vi "Inverter_MAIN.vi"() -> ()   [LabVIEW 2020]
uses:
  controls/INV_test results.ctl
  controls/Inverter_step_type.ctl
  MPB/controls/test control_bools.ctl
  MPB/controls/from_PLC.ctl
  MPB/controls/to_PLC.ctl
  MPB/controls/test_control.ctl
  controls/Inverter_step_array.ctl
  controls/Inverter_step.ctl
  MPB/controls/data type.ctl
  MPB/controls/write_read.ctl
  Hardware Drivers/Keysight E3633 DC PS/dc ps control.ctl
  3b758781-4fb9-4e00-a9b5-a1315665c223.vi
  a98f73de-f23d-4de7-99eb-8fa248b25b7f.vi
panel:
  in  "Test Station":T1
  in  "PLC":T2
  in  "test control":T3
  out "test results":T4={"test pass"=FALSE, "step_type"=enum."prompt", "value"=0.0, "step description"="", "error"={"status"=FALSE, "code"=0, "source"=""}, "save results"=FALSE}
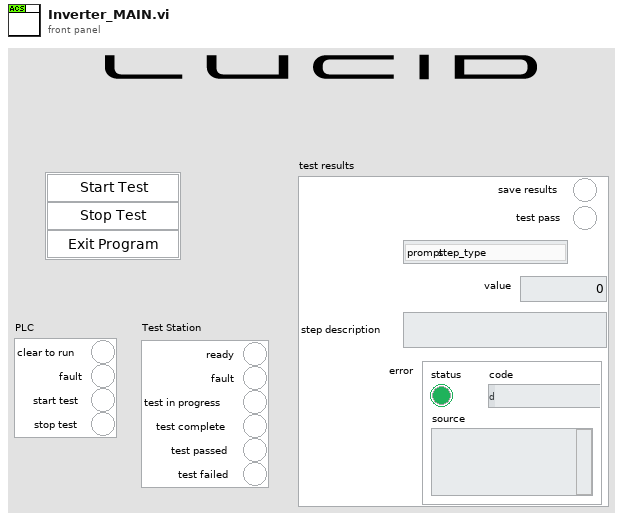
[diagram p1: front panel]
types:
  T1 = typedef "to_PLC.ctl" = cluster{"ready":bool, "fault":bool, "test in progress":bool, "test complete":bool, "test passed":bool, "test failed":bool}
  T2 = typedef "from_PLC.ctl" = cluster{"clear to run":bool, "fault":bool, "start test":bool, "stop test":bool}
  T3 = typedef "test control_bools.ctl" = cluster{"Exit Program":bool, "Stop Test":bool, "Start Test":bool}
  T4 = typedef "INV_test results.ctl" = cluster{"test pass":bool, "step_type":T5, "value":dbl, "step description":string, "error":errorcluster, "save results":bool}
  T5 = typedef "Inverter_step_type.ctl" = enum16{"default", "prompt", "init_12V_power_supply", "12V_power supply on_off", "write_PLC", "read_PLC", "DAQ_Read", "DAQ_Write", "run .bat file", "display_version", "set flow rate", "init_chroma", "set_chroma_V", "set_chroma_ramp", "wait (sec)", "end_test", "record_pass_fail"}
  T6 = typedef "test_control.ctl" = enum16{"Start Test", "Stop Test", "Ready", "Exit Program"}
  T7 = typedef "Inverter_step_array.ctl" = T8[]
  T8 = typedef "Inverter_step.ctl" = cluster{"step_description (prompt)":string, "save results":bool, "step_type":T5, "Step_name":string, "bool":bool[], "data_unit":T9, "dbl":dbl[], "I32":i32[], "string":string[]}
  T9 = typedef "data type.ctl" = enum16{"bool", "string", "I32", "DBL"}
  T10 = cluster{"queue out":refnum<queue>, "queue out":refnum<queue>, "queue out":refnum<queue>}
  T11 = cluster{"Inverter Step Array":T7, "error constant":errorcluster}
  T12 = typedef "dc ps control.ctl" = enum16{"init", "config output", "config OVP", "config current limit", "output on_off", "read output", "self test", "close"}
  T13 = typedef "write_read.ctl" = enum16{"write", "read"}
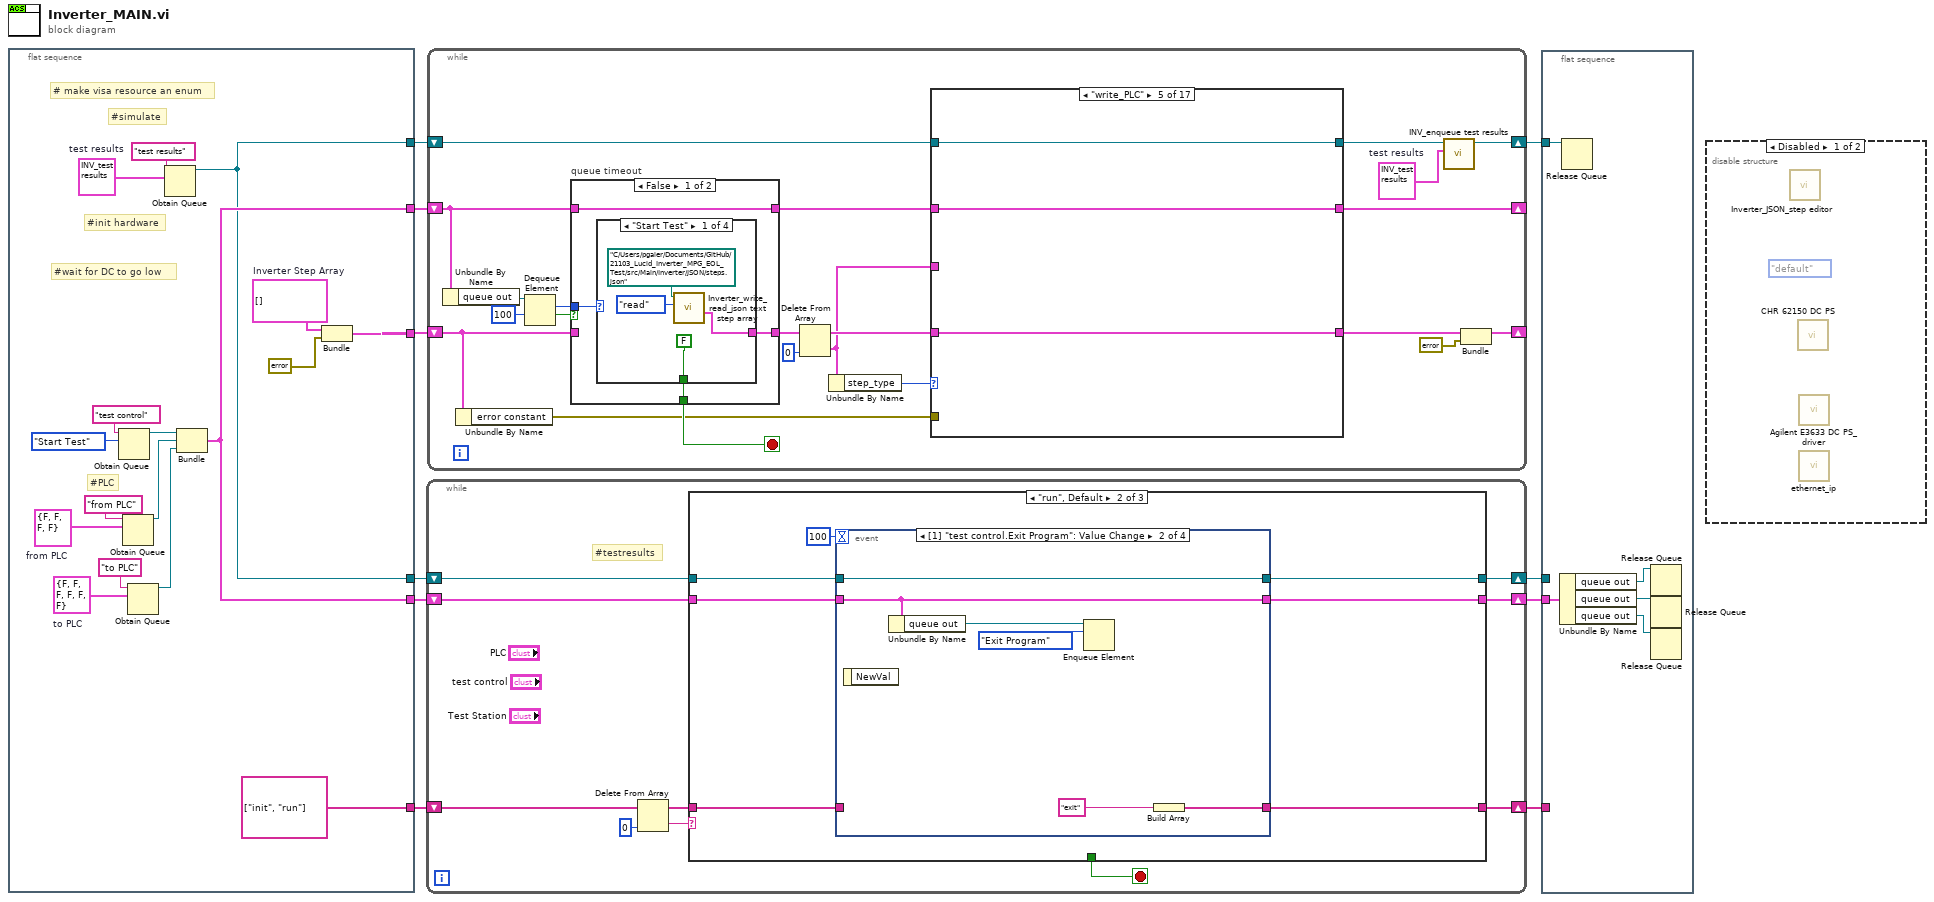
[diagram p0: block diagram]
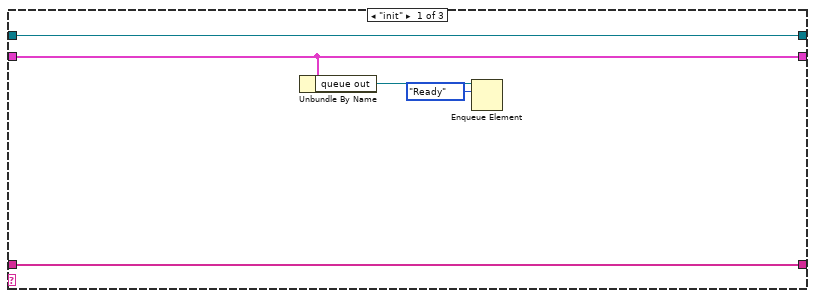
[diagram p3: hidden frame]
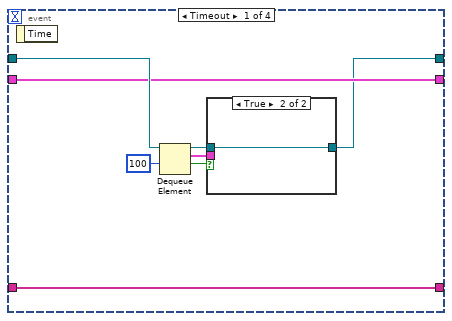
[diagram p4: hidden frame]
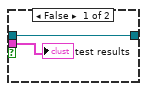
[diagram p5: hidden frame]
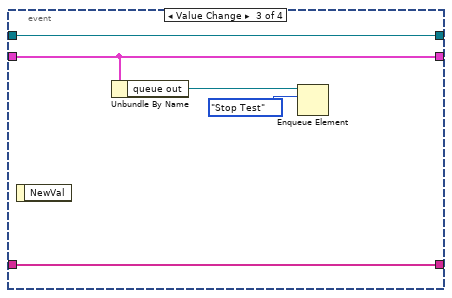
[diagram p6: hidden frame]
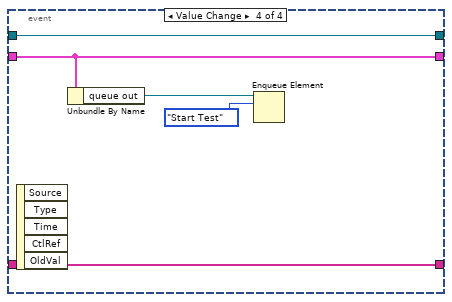
[diagram p7: hidden frame]
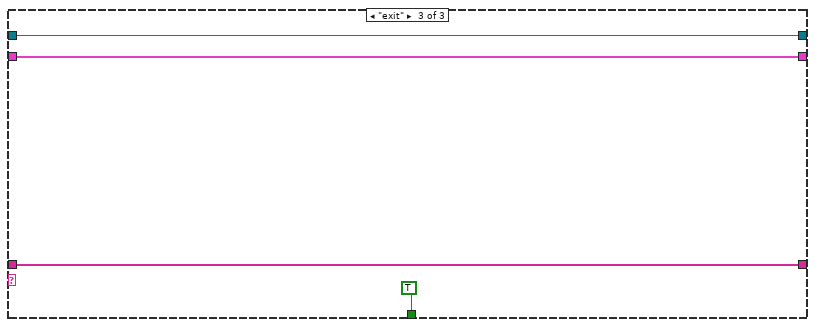
[diagram p8: hidden frame]
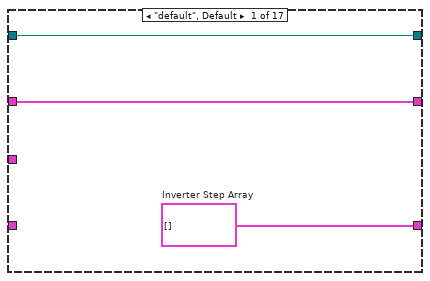
[diagram p9: hidden frame]
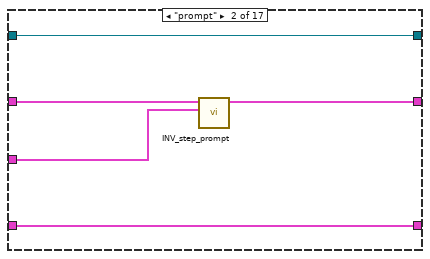
[diagram p10: hidden frame]
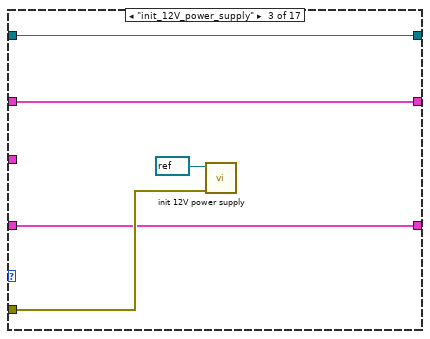
[diagram p11: hidden frame]
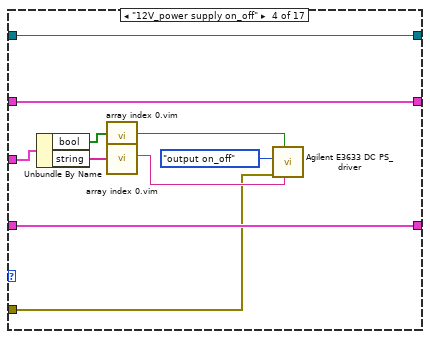
[diagram p12: hidden frame]
diagram:
  n1 = flat-sequence {
    tunnel: [w14] -> w10
    tunnel: [string[] ["init", "run"]] -> w9
    tunnel: [w15] -> w8
    tunnel: [w15] -> w7
    tunnel: [w22] -> w6
    tunnel: [w22] -> w5
    frame #0 {
      w11 = T7 []  # Inverter Step Array
      w23 = T1 {"ready"=FALSE, "fault"=FALSE, "test in progress"=FALSE, "test complete"=FALSE, "test passed"=FALSE, "test failed"=FALSE}  # to PLC
      w24 = T2 {"clear to run"=FALSE, "fault"=FALSE, "start test"=FALSE, "stop test"=FALSE}  # from PLC
      w26 = T4 {"test pass"=FALSE, "step_type"=enum."prompt", "value"=0.0, "step description"="", "error"={"status"=FALSE, "code"=0, "source"=""}, "save results"=FALSE}  # test results
      # "#init hardware"
      # "#wait for DC to go low"
      # "#PLC"
      # "#simulate"
      # "# make visa resource an enum"
      n2 = Obtain Queue(name (unnamed)="test control", element data type=test_control."Start Test" ("test control")) -> (queue out=w25:refnum<queue>)  [unwired: 3 in, 2 out]
      n3 = Obtain Queue(name (unnamed)="from PLC", element data type=w24) -> (queue out=w17:refnum<queue>)  [unwired: 3 in, 2 out]
      n4 = Obtain Queue(name (unnamed)="to PLC", element data type=w23) -> (queue out=w16:refnum<queue>)  [unwired: 3 in, 2 out]
      n5 = Obtain Queue(name (unnamed)="test results", element data type=w26) -> (queue out=w15:refnum<queue>)  [unwired: 3 in, 2 out]
      n6 = Bundle("queue out"=w25, "queue out"=w17, "queue out"=w16) -> (w22:T10)  [unwired: 1 in]
      n7 = Bundle("Inverter Step Array"=w11, "error constant"=errorcluster {"status"=FALSE, "code"=0, "source"=""}) -> (w14:T11)  [unwired: 1 in]
    }
  }
  n8 = while {
    shift-right: [w34] -> w4
    shift-left: w9 -> [w36]
    shift-right: [w29] -> w3
    shift-left: w7 -> [w32]
    shift-right: [w28] -> w2
    shift-left: w6 -> [w31]
    stop <- w30 stop-if-true
    # "#testresults"
    n9 = Delete From Array(array=w36, index=0) -> (deleted portion=w35:string, array with subset deleted=w33:string[])  [unwired: 1 in]
    n10 = case shown="\"run\", Default" w35 {
      tunnel: [w42 w49 w80] -> w34
      tunnel: w33 -> [w42 w48 w80]
      tunnel: w32 -> [w41 w47 w79]
      tunnel: w31 -> [w39 w46 w78]
      tunnel: [_ _ TRUE] -> w30
      tunnel: [w41 w45 w79] -> w29
      tunnel: [w39 w44 w78] -> w28
      frame "init" {
        n11 = Unbundle By Name(w39) -> ("queue out"=w38:refnum<queue>)
        n12 = Enqueue Element(queue=w38, element=test_control."Ready" ("test control")) -> ()  [unwired: 2 in, 3 out]
      }
      frame "run", Default {
        n13 = event shown="[1] \"test control.Exit Program\": Value Change" {
          selector: _ -> [_ _ _ _]
          dyn-events: _ -> [_ _ _ _]
          timeout: 100 -> [_ _ _ _]
          tunnel: w48 -> [w57 _ w71 w76]
          tunnel: [w57 w64 w71 w76] -> w49
          tunnel: w47 -> [w56 w66 w70 w75]
          tunnel: w46 -> [w55 w61 w67 w72]
          tunnel: [w52 w66 w70 w75] -> w45
          tunnel: [w55 w61 w67 w72] -> w44
          event Timeout {
            n14 = event-data() -> ()  [unwired: 1 in, 1 out]
            n15 = Dequeue Element(queue=w56, timeout in ms (-1)=100) -> (queue out=w53:refnum<queue>, element=w50:T4, timed out?=w51:bool)  [unwired: 1 in, 1 out]
            n16 = case shown="True" w51 {
              tunnel: w53 -> [w59 w60]
              tunnel: [w59 w60] -> w52
              tunnel: w50 -> [w58 _]
              frame False {
                "test results" <- w58
              }
              frame True {
              }
            }
          }
          event Value Change {
            n17 = event-data() -> ()  [unwired: 1 in, 1 out]
            n18 = Unbundle By Name(w61) -> ("queue out"=w63:refnum<queue>)
            n19 = Enqueue Element(queue=w63, element=test_control."Exit Program" ("test control")) -> ()  [unwired: 2 in, 3 out]
            n20 = Build Array("exit") -> (w64:string[])
          }
          event Value Change {
            n21 = event-data() -> ()  [unwired: 1 in, 1 out]
            n22 = Unbundle By Name(w67) -> ("queue out"=w69:refnum<queue>)
            n23 = Enqueue Element(queue=w69, element=test_control."Stop Test" ("test control")) -> ()  [unwired: 2 in, 3 out]
          }
          event Value Change {
            n24 = event-data() -> ()  [unwired: 1 in, 5 out]
            n25 = Unbundle By Name(w72) -> ("queue out"=w74:refnum<queue>)
            n26 = Enqueue Element(queue=w74, element=test_control."Start Test" ("test control")) -> ()  [unwired: 2 in, 3 out]
          }
        }
      }
      frame "exit" {
      }
    }
  }
  n27 = while {
    shift-right: [w94] -> _
    shift-left: w10 -> [w93]
    shift-right: [w81] -> w1
    shift-left: w8 -> [w91]
    shift-right: [w88] -> _
    shift-left: w5 -> [w95]
    stop <- w99 stop-if-true
    w83 = T4 {"test pass"=FALSE, "step_type"=enum."prompt", "value"=0.0, "step description"="", "error"={"status"=FALSE, "code"=0, "source"=""}, "save results"=FALSE}  # test results
    n28 = Unbundle By Name(w95) -> ("queue out"=w102:refnum<queue>)
    n29 = Unbundle By Name(w93) -> ("error constant"=w84:errorcluster)
    n30 = Dequeue Element(queue=w102, timeout in ms (-1)=100) -> (element=w100:T6, timed out?=w101:bool)  [unwired: 1 in, 2 out]
    n31 = case "queue timeout" shown="False" w101 {
      tunnel: w93 -> [_ w180]
      tunnel: [w165 w179] -> w97
      tunnel: w100 -> [w168 _]
      tunnel: [w167 FALSE] -> w99
      tunnel: w95 -> [w166 w182]
      tunnel: [w166 w182] -> w89
      frame False {
        n32 = case shown="\"Start Test\"" w168 {
          tunnel: [FALSE FALSE FALSE TRUE] -> w167
          tunnel: [w169 w173 w175 w177] -> w165
          frame "Start Test" {
            n33 = call "Inverter_write_read_json text step array.vi"("write_read"=write_read."read", "File Path"=path "C:/Users/pgaier/Documents/GitHub/21103_Lucid_Inverter_MPG_EOL_Test/src/Main/Inverter/JSON/steps.json") -> ("steps array out"=w169:T8[])  [unwired: 7 in, 2 out]
          }
          frame "Stop Test" {
            w173 = T7 []  # Inverter Step Array
          }
          frame "Ready", Default {
            w175 = T7 []  # Inverter Step Array
          }
          frame "Exit Program" {
            w177 = T7 []  # Inverter Step Array
          }
        }
      }
      frame True {
        n34 = Unbundle By Name(w180) -> ("Inverter Step Array"=w179:T7)
      }
    }
    n35 = Delete From Array(array=w97, index=0) -> (deleted portion=w85:T8, array with subset deleted=w87:T7)  [unwired: 1 in]
    n36 = Unbundle By Name(w85) -> ("step_type"=w90:T5)
    n37 = case shown="\"write_PLC\"" w90 {
      tunnel: w91 -> [w105 w110 w113 w125 w128 w131 w134 w137 w140 w143 w146 w149 w152 w155 w158 w161 w164]
      tunnel: [w105 w110 w113 w125 w128 w131 w134 w137 w140 w143 w146 w149 w152 w155 w158 w161 w164] -> w82
      tunnel: w89 -> [w104 w109 w111 w124 w127 w130 w133 w136 w139 w142 w145 w148 w151 w154 w157 w160 w163]
      tunnel: [w104 w107 w111 w124 w127 w130 w133 w136 w139 w142 w145 w148 w151 w154 w157 w160 w163] -> w88
      tunnel: w87 -> [_ w108 w112 w123 w126 w129 w132 w135 w138 w141 w144 w147 w150 w153 w156 w159 _]
      tunnel: [w103 w108 w112 w123 w126 w129 w132 w135 w138 w141 w144 w147 w150 w153 w156 w159 w162] -> w86
      tunnel: w85 -> [_ w106 _ w122 _ _ _ _ _ _ _ _ _ _ _ _ _]
      tunnel: w84 -> [_ _ w114 w116 _ _ _ _ _ _ _ _ _ _ _ _ _]
      frame "default", Default {
        w103 = T7 []  # Inverter Step Array
      }
      frame "prompt" {
        n38 = call "INV_step_prompt.vi"("step"=w106, "Cluster in"=w109) -> ("Cluster out"=w107:T10)  [unwired: 7 in, 2 out]
      }
      frame "init_12V_power_supply" {
        n39 = call "init 12V power supply.vi"("error in"=w114, "VISA Refnum in"=refnum<visa-resource-name> refnum ("VISA resource in")) -> ()  [unwired: 9 in, 1 out]
      }
      frame "12V_power supply on_off" {
        n40 = Unbundle By Name(w122) -> ("bool"=w118:bool[], "string"=w121:string[])
        n41 = call "array index 0.vim"("32INT in"=w118) -> ("Numeric"=w117:bool)  [unwired: 10 in]
        n42 = call "array index 0.vim"("32INT in"=w121) -> ("Numeric"=w119:string)  [unwired: 10 in]
        n43 = call "Agilent E3633 DC PS_driver.vi"("VISA resource in"=w119, "Enable Output (T: Enable)"=w117, "Error In"=w116, "agilent E3633 DC PS"=dc_ps_control."output on_off") -> ()  [unwired: 4 in, 4 out]
      }
      frame "write_PLC" {
      }
      frame "read_PLC" {
      }
      frame "wait (sec)" {
      }
      frame "record_pass_fail" {
      }
      frame "DAQ_Read" {
      }
      frame "DAQ_Write" {
      }
      frame "run .bat file" {
      }
      frame "display_version" {
      }
      frame "set flow rate" {
      }
      frame "init_chroma" {
      }
      frame "set_chroma_V" {
      }
      frame "set_chroma_ramp" {
      }
      frame "end_test" {
        w162 = T7 []  # Inverter Step Array
      }
    }
    n44 = call "INV_enqueue test results.vi"("test results"=w83, "queue in"=w82) -> ("queue out"=w81:refnum<queue>)  [unwired: 8 in, 1 out]
    n45 = Bundle("Inverter Step Array"=w86, "error constant"=errorcluster {"status"=FALSE, "code"=0, "source"=""}) -> (w94:T11)  [unwired: 1 in]
  }
  n46 = flat-sequence {
    tunnel: w4 -> [_]
    tunnel: w3 -> [_]
    tunnel: w2 -> [w187]
    tunnel: w1 -> [w183]
    frame #0 {
      n47 = Unbundle By Name(w187) -> ("queue out"=w186:refnum<queue>, "queue out"=w185:refnum<queue>, "queue out"=w184:refnum<queue>)
      n48 = Release Queue(queue=w183) -> ()  [unwired: 2 in, 3 out]
      n49 = Release Queue(queue=w186) -> ()  [unwired: 2 in, 3 out]
      n50 = Release Queue(queue=w185) -> ()  [unwired: 2 in, 3 out]
      n51 = Release Queue(queue=w184) -> ()  [unwired: 2 in, 3 out]
    }
  }
  n52 = disable-structure shown="Disabled" {
    frame Disabled {
      (unwired) Inverter_step_type."default" ("step_type")
      n53 = call "Inverter_JSON_step editor.vi"() -> ()  [unwired: 12 in]
      n54 = call "CHR 62150 DC PS.vi"() -> ()  [unwired: 12 in]
      n55 = call "Agilent E3633 DC PS_driver.vi"() -> ()  [unwired: 8 in, 4 out]
      n56 = call "ethernet_ip.vi"() -> ()  [unwired: 7 in, 9 out]
    }
    frame Enabled {
    }
  }
